vi "DataLog.vi"(4 "CH2 SP":dbl, 6 "CH1 SP":dbl, 8 "error in (no error)":errorcluster, 9 "CH2":dbl, 10 "CH1":dbl, 11 "Controller Name":string="F4") -> (0 "error out":errorcluster)   [LabVIEW 2010]
doc: "Use this template to build a VI to use as a subVI."
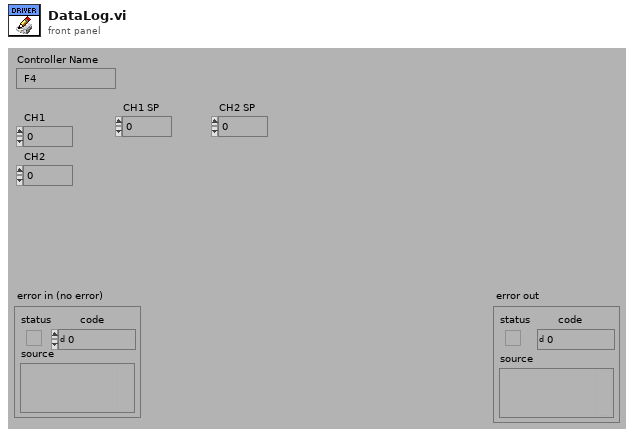
[diagram p1: front panel]
types:
  T1 = enum16{"open", "open or create", "create or replace", "create", "open (read-only)"}
  T2 = typedef "Path InitPaths__FS.ctl" = cluster{"Ctrller CFG":path, "INI":path, "Profile":path, "EventLog":path, "Data":path}
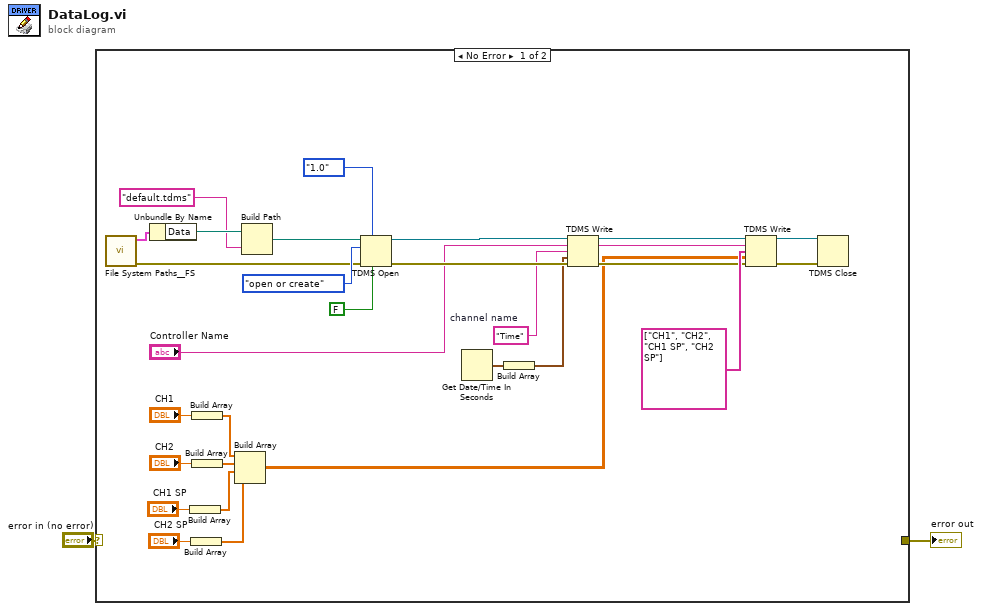
[diagram p0: block diagram]
diagram:
  n1 = case shown="No Error" "error in (no error)" {
    selector: "error in (no error)" -> [_ w32]
    tunnel: [_ w32] -> w1
    frame No Error {
      w23 = "Time"  # channel name
      n2 = call "File System Paths__FS.vi"() -> ("error out"=w9:errorcluster, "FilePaths"=w13:T2)  [unwired: 9 in, 1 out]
      n3 = Unbundle By Name(w13) -> ("Data"=w12:path)
      n4 = Build Array("CH1 SP") -> (w4:dbl[])
      n5 = Build Array("CH2 SP") -> (w3:dbl[])
      n6 = Build Array("CH1") -> (w17:dbl[])
      n7 = Build Array("CH2") -> (w16:dbl[])
      n8 = Build Array(w17, w16, w4, w3) -> (w18:dbl[][])
      n9 = Build Path(base path=w12, name or relative path="default.tdms") -> (appended path=w10:path)
      n10 = TDMS Open(6:FALSE ("disable buffering (T)"), 7:enum16{"1.0", "2.0"}."1.0" ("file format version (2.0)"), 8:w9, 10:T1."open or create" ("operation"), 11:w10) -> (0:w27:errorcluster, 3:w28:refnum<k34>)  [unwired: 1 in]
      n11 = Get Date/Time In Seconds() -> (seconds since 1Jan1904=w22:timestamp)
      n12 = Build Array(w22) -> (w21:timestamp[])
      n13 = TDMS Write(0:w28, 5:"Controller Name", 7:w23, 9:w21, 11:w27) -> (4:w20:refnum<k34>, 6:w7:string, 15:w19:errorcluster)  [unwired: 1 in, 1 out]
      n14 = TDMS Write(0:w20, 5:w7, 7:string[] ["CH1", "CH2", "CH1 SP", "CH2 SP"] ("channel name(s) in (Untitled)"), 9:w18, 11:w19) -> (4:w31:refnum<k34>, 15:w30:errorcluster)  [unwired: 1 in, 2 out]
      n15 = TDMS Close(8:w30, 11:w31) -> ()  [unwired: 2 out]
    }
    frame Error {
    }
  }
  "error out" <- w1
